vi "Write Chnl.vi"(8 "error in (no error)":errorcluster, 10 "BME_DG_Chnl":refnum<class "BME_DG_Chnl.lvclass">, 11 "BME_DG_Base in":refnum<class "BME_DG_Base.lvclass">) -> (0 "error out":errorcluster, 3 "BME_DG_Base out":refnum<class "BME_DG_Base.lvclass">)   [LabVIEW 2009, in "POLARIS BME DG.lvlib" / "BME_DG_Base.lvclass"]
uses:
  BME_DG_Base.lvclass
  BME_DG_Chnl/BME_DG_Chnl.lvclass
  BME_DG_Base.lvclass/BME_DG_Base.ctl
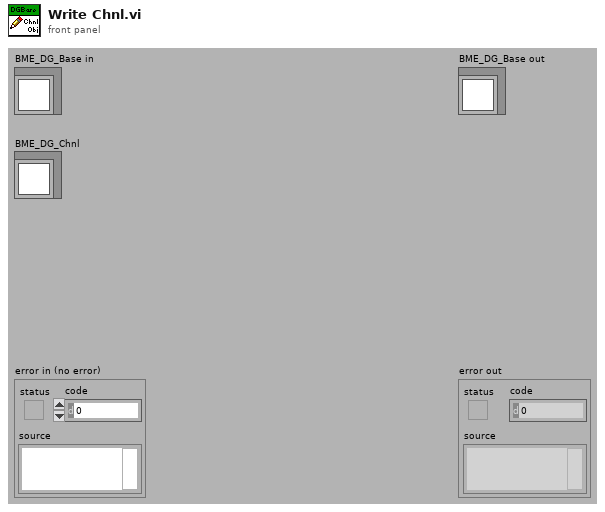
[diagram p1: front panel]
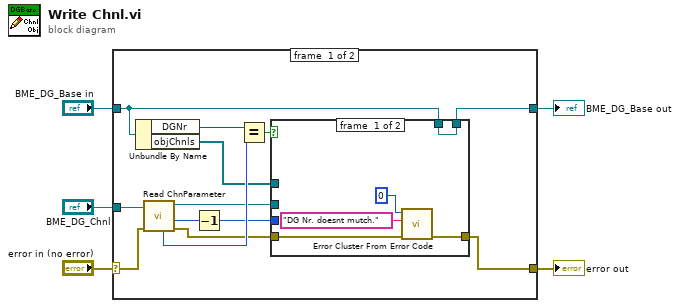
[diagram p0: block diagram]
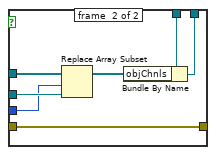
[diagram p2: hidden frame]
diagram:
  n1 = case shown="No Error" "error in (no error)" {
    selector: "error in (no error)" -> [w8 w32]
    tunnel: [w6 w32] -> w4
    tunnel: [w9 w31] -> w2
    tunnel: "BME_DG_Base in" -> [w10 w31]
    tunnel: "BME_DG_Chnl" -> [w18 _]
    frame #0 {
      n2 = Unbundle By Name(w10) -> ("DGNr"=w17:i32, "objChnls"=w15:refnum<class "BME_DG_Chnl.lvclass">[])
      n3 = call-dynamic "Read ChnParameter.vi"("error in (no error)"=w8, "BME_DG_Chnl in"=w18) -> ("error out"=w7:errorcluster, "Nr"=w13:i32, "BME_DG_Chnl out"=w14:refnum<class "BME_DG_Chnl.lvclass">, "DG Nr"=w16:i32)  [unwired: 4 in, 2 out]
      n4 = Decrement(x=w13) -> (x-1=w12:i32)
      n5 = Equal?(x=w17, y=w16) -> (x = y?=w11:bool)
      n6 = case shown="False" w11 {
        tunnel: w15 -> [_ w30]
        tunnel: w14 -> [_ w29]
        tunnel: w12 -> [_ w28]
        tunnel: w10 -> [w23 w27]
        tunnel: [w23 w25] -> w9
        tunnel: w7 -> [w22 w24]
        tunnel: [w21 w24] -> w6
        frame #0 {
          n7 = call <vilib>:"Error Cluster From Error Code.vi"("error in (no error)"=w22, "error message (\"\")"="DG Nr. doesnt mutch." ("error message (\"\")"), "error code (0)"=0) -> ("error out"=w21:errorcluster)  [unwired: 6 in]
        }
        frame #1 {
          n8 = Replace Array Subset(array=w30, new element=w29, index=w28) -> (w26:refnum<class "BME_DG_Chnl.lvclass">[])
          n9 = Bundle By Name(cluster=w27, "objChnls"=w26) -> (w25:refnum<class "BME_DG_Base.lvclass">)
        }
      }
    }
    frame #1 {
    }
  }
  "error out" <- w4
  "BME_DG_Base out" <- w2
